vi "wSetup.vi"(0 "Socket in":refnum<class "Socket.lvclass">, 5 "IP Address":string, 7 "Port":u16, 11 "error in (no error)":errorcluster) -> (4 "Socket out":refnum<class "Socket.lvclass">, 15 "error out":errorcluster)   [LabVIEW 2011, in "Socket.lvclass"]
uses:
  Socket.lvclass
  Socket.lvclass/Socket.ctl
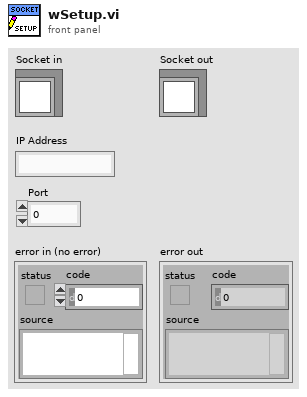
[diagram p1: front panel]
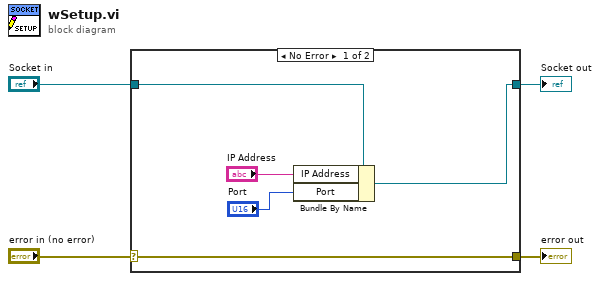
[diagram p0: block diagram]
diagram:
  n1 = case shown="No Error" "error in (no error)" {
    selector: "error in (no error)" -> [w9 w10]
    tunnel: [w9 w10] -> w3
    tunnel: [w7 w11] -> w1
    tunnel: "Socket in" -> [w8 w11]
    frame No Error {
      n2 = Bundle By Name(cluster=w8, "IP Address"="IP Address", "Port"="Port") -> (w7:refnum<class "Socket.lvclass">)
    }
    frame Error {
    }
  }
  "error out" <- w3
  "Socket out" <- w1
